vi "FlexDDS-NG_DCP_WriteDRL.vi"(6 "Ramp type":enum32{"Frequency", "Phase", "Amplitude"}(ring), 7 "mirror frequency?":bool, 8 "low limit":dbl format="%#_6f", 9 "high limit":dbl=1.0 format="%#_6f", 10 "Channels":T1(ring)=enum."Both channels", 11 "initial instruction string":string) -> (3 "appended instruction string":string="dcp spi:DRL=0xFFFC000000000000\r")   [LabVIEW 2016]
panel:
  # "NOTE: Limit depends on ramp type:\nFrequency: in Hz\nAmplitude: in unit 0..1\nPhase: in degrees (0..360)"
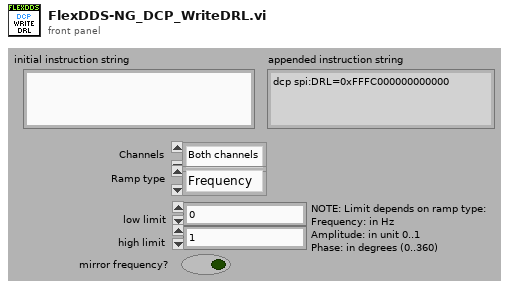
[diagram p1: front panel]
types:
  T1 = enum32{"Channel 0", "Channel 1", "Both channels"}
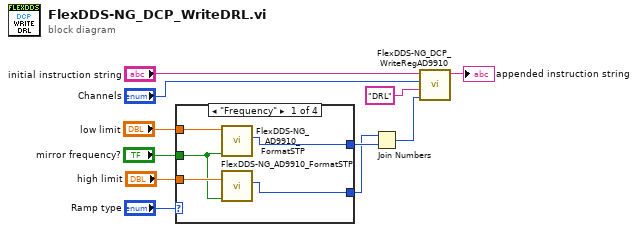
[diagram p0: block diagram]
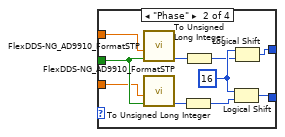
[diagram p2: hidden frame]
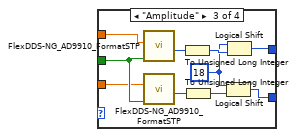
[diagram p3: hidden frame]
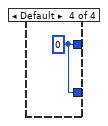
[diagram p4: hidden frame]
diagram:
  n1 = case shown="\"Frequency\"" "Ramp type" {
    tunnel: "low limit" -> [w16 w25 w34 _]
    tunnel: "high limit" -> [w15 w24 w35 _]
    tunnel: "mirror frequency?" -> [w14 w26 w36 _]
    tunnel: [w13 w18 w31 w37] -> w1
    tunnel: [w12 w17 w27 w37] -> w2
    frame "Frequency" {
      n2 = call "FlexDDS-NG_AD9910_FormatSTP.vi"("mirror frequency?"=w14, "frequency Hz (0..400M)"=w16) -> ("frequency tuning word (FTW) out"=w12:u32)  [unwired: 6 in, 3 out]
      n3 = call "FlexDDS-NG_AD9910_FormatSTP.vi"("mirror frequency?"=w14, "frequency Hz (0..400M)"=w15) -> ("frequency tuning word (FTW) out"=w13:u32)  [unwired: 6 in, 3 out]
    }
    frame "Phase" {
      w21 = u32 16 ("x")
      n4 = call "FlexDDS-NG_AD9910_FormatSTP.vi"("mirror frequency?"=w26, "phase degrees (0..360)"=w25) -> ("phase offset word (POW) out"=w23:u16)  [unwired: 6 in, 3 out]
      n5 = call "FlexDDS-NG_AD9910_FormatSTP.vi"("mirror frequency?"=w26, "phase degrees (0..360)"=w24) -> ("phase offset word (POW) out"=w22:u16)  [unwired: 6 in, 3 out]
      n6 = To Unsigned Long Integer(number=w22) -> (unsigned 32bit integer=w19:u32)
      n7 = To Unsigned Long Integer(number=w23) -> (unsigned 32bit integer=w20:u32)
      n8 = Logical Shift(y=w21, x=w19) -> (x << y=w18:u32)
      n9 = Logical Shift(y=w21, x=w20) -> (x << y=w17:u32)
    }
    frame "Amplitude" {
      w28 = u32 18 ("x")
      n10 = call "FlexDDS-NG_AD9910_FormatSTP.vi"("mirror frequency?"=w36, "amplitude (0..1)"=w34) -> ("amplitude scale factor (ASF) out"=w32:u16)  [unwired: 6 in, 3 out]
      n11 = call "FlexDDS-NG_AD9910_FormatSTP.vi"("mirror frequency?"=w36, "amplitude (0..1)"=w35) -> ("amplitude scale factor (ASF) out"=w33:u16)  [unwired: 6 in, 3 out]
      n12 = To Unsigned Long Integer(number=w32) -> (unsigned 32bit integer=w29:u32)
      n13 = To Unsigned Long Integer(number=w33) -> (unsigned 32bit integer=w30:u32)
      n14 = Logical Shift(y=w28, x=w30) -> (x << y=w31:u32)
      n15 = Logical Shift(y=w28, x=w29) -> (x << y=w27:u32)
    }
    frame Default {
      w37 = u32 0 ("frequency tuning word (FTW) out")
    }
  }
  n16 = Join Numbers(hi=w1, lo=w2) -> ((hi.lo)=w3:u64)
  n17 = call "FlexDDS-NG_DCP_WriteRegAD9910.vi"("register content"=w3, "AD9910 register name"="DRL" ("format string"), "Channels"="Channels", "initial instruction string"="initial instruction string") -> ("appended instruction string"=→"appended instruction string":string)  [unwired: 7 in]
